vi "RT DO FGV.vi"(7 "Enum":T1, 9 "Start Time":timestamp, 10 "DO Channel Names":string[](array[string]), 11 "DO in":bool[](array[boolean])) -> (1 "DO Waveform":waveform(dbl)[](array[waveform]), 2 "DO Names Out":string[](array[string]), 3 "DO out":bool[](array[boolean]))   [LabVIEW 2022 SP3]
uses:
  RT Controls/DO FGV.ctl
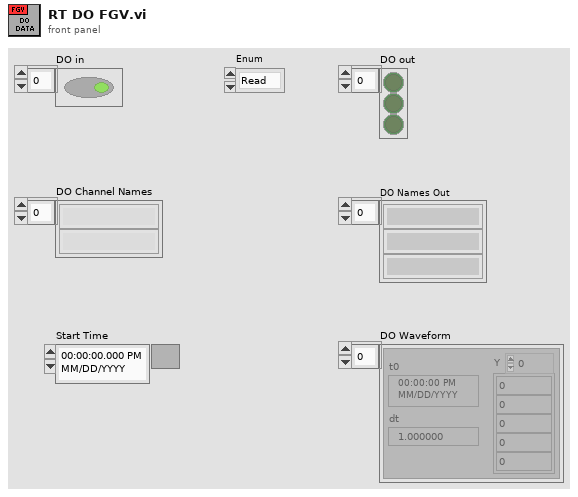
[diagram p1: front panel]
types:
  T1 = typedef "DO FGV.ctl" = enum16{"Read", "Write", "Start time", "init", "Read only"}
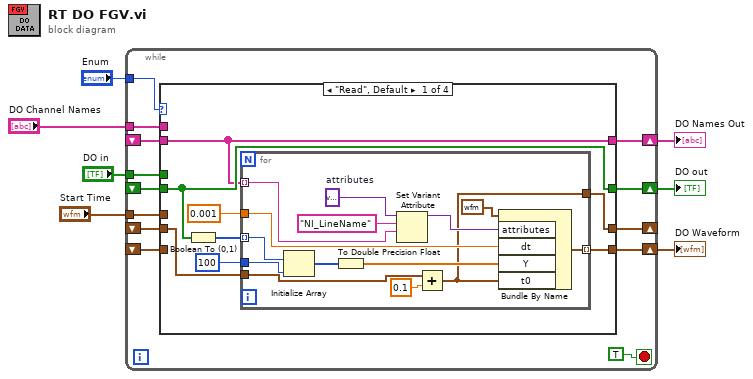
[diagram p0: block diagram]
diagram:
  n1 = while {
    tunnel: "Enum" -> [w19]
    tunnel: "DO in" -> [w18]
    shift-right: [w17] -> w3
    shift-left: _ -> [w16]
    tunnel: "Start Time" -> [w15]
    shift-right: [w14] -> _
    shift-left: _ -> [w13]
    shift-right: [w12] -> w4
    shift-left: _ -> [w11]
    shift-right: [w9] -> w1
    shift-left: _ -> [w10]
    tunnel: "DO Channel Names" -> [w8]
    stop <- TRUE stop-if-true
    n2 = case shown="\"Read\", Default" w19 {
      tunnel: w18 -> [_ w46 _ _]
      tunnel: [w25 w46 w48 w53] -> w17
      tunnel: w16 -> [w25 _ w48 w53]
      tunnel: w15 -> [_ _ w50 _]
      tunnel: [w22 w45 w50 w52] -> w14
      tunnel: w13 -> [w21 w45 _ w52]
      tunnel: [w24 w44 w49 w51] -> w12
      tunnel: w11 -> [_ w44 w49 w51]
      tunnel: w10 -> [w23 w43 _ w54]
      tunnel: [w23 w43 w47 w54] -> w9
      tunnel: w8 -> [_ _ w47 _]
      frame "Read", Default {
        n3 = Boolean To (0,1)(Boolean=w25) -> (0, 1=w27:i16[])
        n4 = for {
          tunnel: w27 -> [w41] mode=indexing
          tunnel: [w42] -> w24 mode=indexing
          tunnel: 100 ("Size") -> [w38]
          tunnel: w23 -> [w36] mode=indexing
          tunnel: 0.001 ("dt(sec)") -> [w33]
          tunnel: [w29] -> w22
          tunnel: w21 -> [w31]
          w37 = variant  # attributes
          n5 = Initialize Array(w41, w38) -> (w40:i16[])
          n6 = To Double Precision Float(number=w40) -> (double precision float=w39:dbl[])
          n7 = Set Variant Attribute(Variant=w37, name="NI_LineName", value=w36) -> (Variant out=w32:variant)  [unwired: 1 in, 2 out]
          n8 = Add(x=w31, y=0.1) -> (x+y=w29:timestamp)
          n9 = Bundle By Name(cluster=waveform(dbl) {"t0"=timestamp(0 s since 1904-01-01), "dt"=1.0, "Y"=[]} ("waveform"), "attributes"=w32, "dt"=w33, "Y"=w39, "t0"=w29) -> (w42:waveform(dbl))
        }
      }
      frame "Write" {
      }
      frame "Start time" {
      }
      frame "Read only" {
      }
    }
  }
  "DO Waveform" <- w4
  "DO out" <- w3
  "DO Names Out" <- w1
